vi "Tuoicaytudong.vi"() -> ()   [LabVIEW 2022 SP3]
uses:
  <vilib>/Instr/_visa.llb/VISA Configure Serial Port (Instr).vi
panel:
  out "Command Controll":string
  out "PUMP":bool
  out "Level (%)":dbl(knob) scale=0.0..100.0
  out "Moisture(%)":dbl(knob) scale=0.0..100.0
  in  "read":bool=TRUE
  in  "flow control":u16(ring) items=["None"=0, "XON/XOFF"=1, "RTS/CTS"=2, "DTR/DSR"=4]
  in  "stop bits":u16(ring)=10 items=["1.0"=10, "1.5"=15, "2.0"=20]
  in  "parity":u16(ring) items=["None", "Odd", "Even", "Mark", "Space"]
  in  "VISA resource name":refnum<visa-resource-name>="COM1"
  in  "baud rate":u32=9600
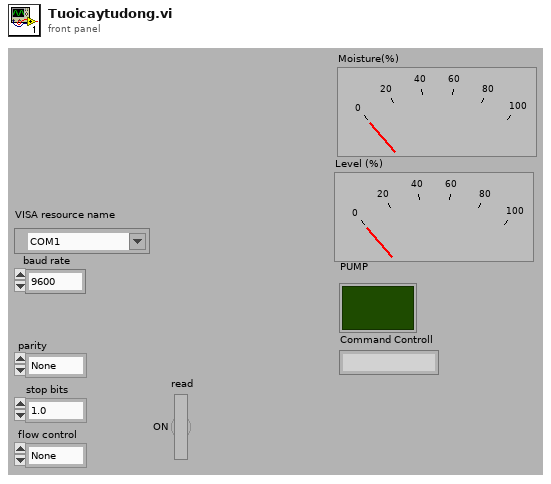
[diagram p1: front panel]
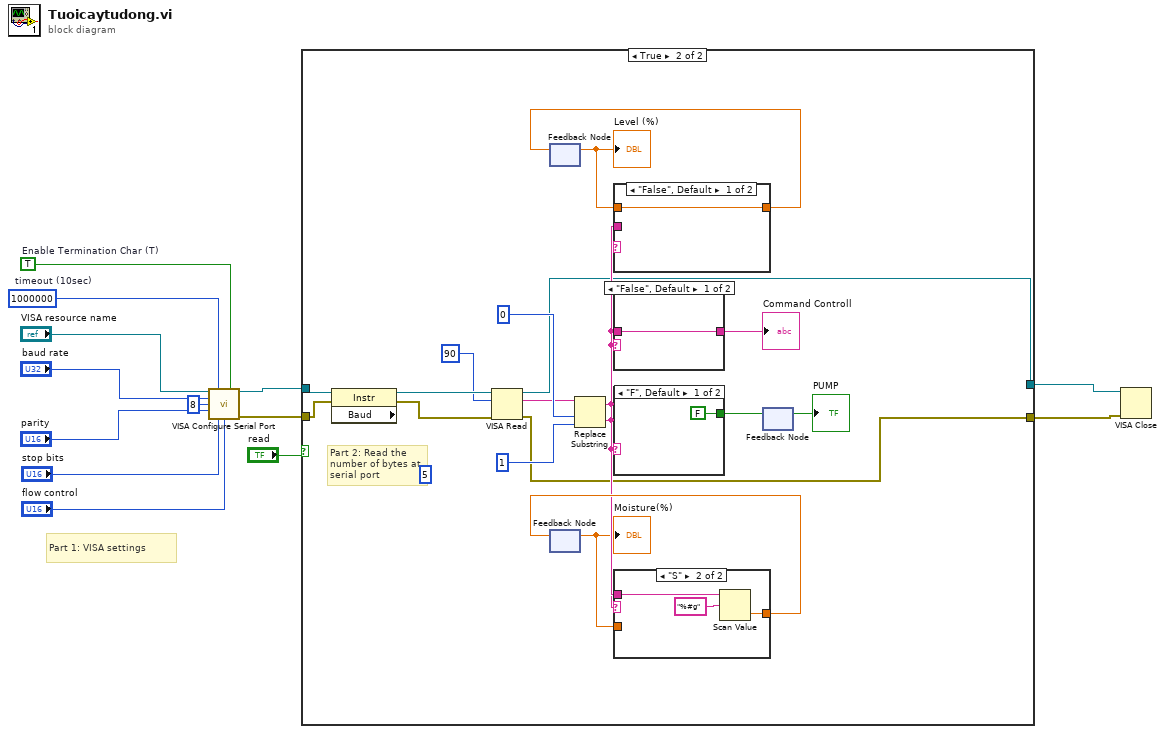
[diagram p0: block diagram]
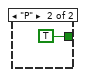
[diagram p4: hidden frame]
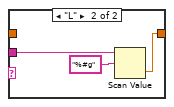
[diagram p5: hidden frame]
diagram:
  w9 = TRUE  # Enable Termination Char (T)
  w10 = u32 1000000  # timeout (10sec)
  # "Part 2: Read the number of bytes at \nserial port"
  # "Part 1: VISA settings"
  n1 = call-poly "VISA Configure Serial Port"("VISA resource name"="VISA resource name", "timeout (10sec)"=w10, "Enable Termination\nChar (T)"=w9, "baud rate (9600)"="baud rate", "data bits (8)"=u16 8, "parity (0:none)"="parity", "stop bits (10: 1 bit)"="stop bits", "flow control (0:none)"="flow control") -> ("VISA resource name out"=w5:refnum<visa-resource-name>, "error out"=w7:errorcluster)  [unwired: 1 in, 5 out]
  n2 = case shown="True" "read" {
    tunnel: w7 -> [w15 w34]
    tunnel: [w15 w20] -> w3
    tunnel: [w14 w21] -> w4
    tunnel: w5 -> [w14 w18]
    frame False {
    }
    frame True {
      (unwired) u32 5 ("bytes read")
      n3 = property class="Instr" props=["Baud"](reference=w18, error in=w34) -> (reference out=w17:refnum<visa-resource-name>, error out=w33:errorcluster)  [unwired: 1 out]
      n4 = VISA Read(VISA resource name=w17, byte count=u32 90, error in (no error)=w33) -> (VISA resource name out=w21:refnum<visa-resource-name>, read buffer=w19:string, error out=w20:errorcluster)  [unwired: 1 out]
      n5 = feedback #1() -> (w26:dbl)  [unwired: 1 in]
      "Level (%)" <- w26
      n6 = feedback #2() -> (w25:dbl)  [unwired: 1 in]
      "Moisture(%)" <- w25
      n7 = Replace Substring(2:1, 3:0, 5:w19) -> (0:w22:string, 1:w28:string)  [unwired: 1 in]
      n8 = case shown="\"False\", Default" w22 {
        tunnel: w28 -> [_ w41]
        tunnel: [w39 w40] -> w29
        tunnel: w26 -> [w39 _]
        frame "False", Default {
        }
        frame "L" {
          n9 = Scan Value(string=w41, format string="%#g") -> (value=w40:dbl)  [unwired: 1 in, 1 out]
        }
      }
      n10 = feedback-in #1(w29) -> ()
      n11 = case shown="\"False\", Default" w22 {
        tunnel: w28 -> [w35 w36]
        tunnel: [w35 w36] -> w27
        frame "False", Default {
        }
        frame "C" {
        }
      }
      "Command Controll" <- w27
      n12 = case shown="\"F\", Default" w22 {
        tunnel: [FALSE TRUE] -> w24
        frame "F", Default {
        }
        frame "P" {
        }
      }
      n13 = case shown="\"S\"" w22 {
        tunnel: w28 -> [_ w46]
        tunnel: [w43 w44] -> w30
        tunnel: w25 -> [w43 _]
        frame "False", Default {
        }
        frame "S" {
          n14 = Scan Value(string=w46, format string="%#g") -> (value=w44:dbl)  [unwired: 1 in, 1 out]
        }
      }
      n15 = feedback-in #2(w30) -> ()
      n16 = feedback #3() -> (→"PUMP":bool)  [unwired: 1 in]
      n17 = feedback-in #3(w24) -> ()
    }
  }
  n18 = VISA Close(VISA resource name=w4, error in (no error)=w3) -> ()  [unwired: 1 out]
